vi "Digital Output DAQ Assistant.vi"() -> ()   [LabVIEW 2020]
panel:
  in  "Array":bool[](array[boolean])
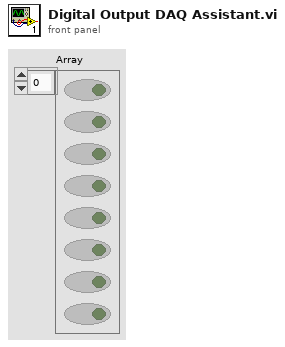
[diagram p1: front panel]
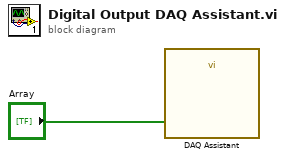
[diagram p0: block diagram]
diagram:
  n1 = call "DAQ Assistant"("data"="Array") -> ()  [unwired: 17 in, 2 out]
